vi "Get Target Info.vi"(11 "error in":errorcluster) -> (4 "Target Found?":bool, 6 "Angle (deg)":dbl, 8 "Distance (in)":dbl, 10 "timestamp":u32, 15 "error out":errorcluster)   [LabVIEW 2016, in "Vision Drive.lvlib"]
uses:
  Vision Drive.lvlib
  Private/Vision Target Global.vi
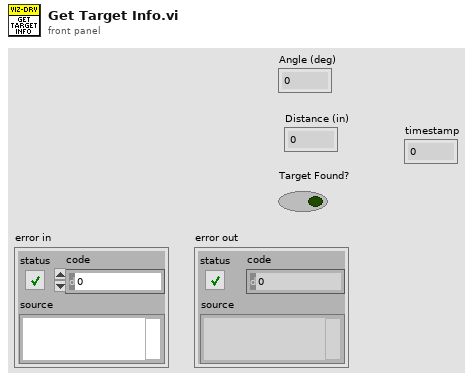
[diagram p1: front panel]
types:
  T1 = typedef "Vision Drive.lvlib/Target to Robot.ctl" = cluster{"Angle (deg)":dbl, "Distance (in)":dbl, "timestamp (ms)":u32, "Target Found":bool}
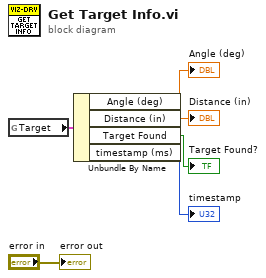
[diagram p0: block diagram]
diagram:
  n1 = global read "Vision Target Global.vi" "Target"() -> (w6:T1)
  n2 = Unbundle By Name(w6) -> ("Angle (deg)"=→"Angle (deg)":dbl, "Distance (in)"=→"Distance (in)":dbl, "Target Found"=→"Target Found?":bool, "timestamp (ms)"=→"timestamp":u32)
  "error out" <- "error in"
